vi "motion control_Z.vi"(2 "position":dbl, 3 "acceleration":dbl, 4 "maxVelocity":dbl, 5 ".NET Refnum in":refnum<k24>) -> (1 ".NET Refnum out":refnum<k24>)   [LabVIEW 2021]
uses:
  C:/Users/User/Documents/Published_files/thorlabs_files/ThorLabs.MotionControl.KCube.DCServoCLI.dll
  thorlabs_files/ThorLabs.MotionControl.KCube.DCServoCLI.dll
  <vilib>/ptbypt/NI_PtbyPt.lvlib
panel:
  out "end":bool=TRUE
  out "x < y?":bool
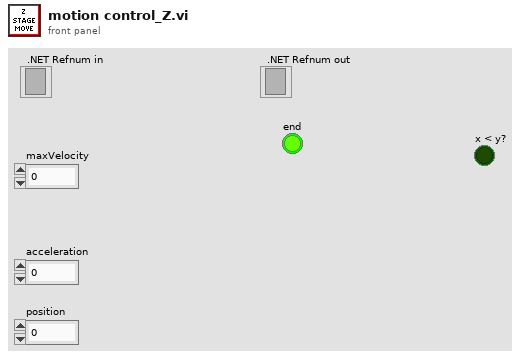
[diagram p1: front panel]
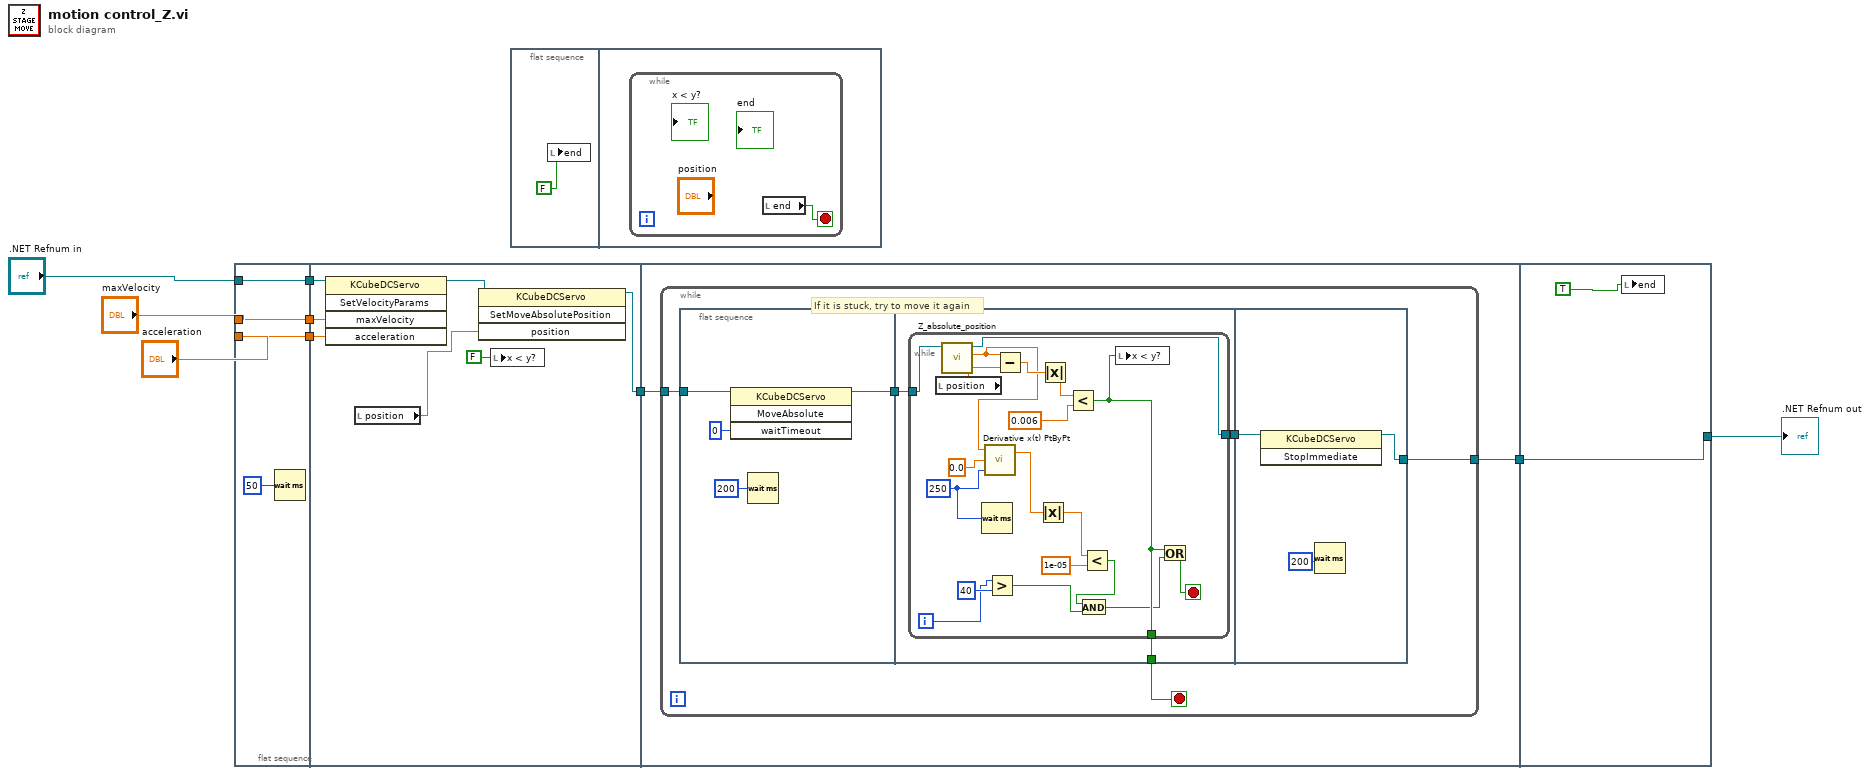
[diagram p0: block diagram]
diagram:
  n1 = flat-sequence {
    tunnel: "maxVelocity" -> [w11]
    tunnel: "acceleration" -> [w12]
    tunnel: ".NET Refnum in" -> [w13]
    tunnel: [w13] -> w3
    tunnel: [w12] -> w2
    tunnel: [w11] -> w1
    tunnel: [w14] -> w6
    tunnel: w3 -> [w20]
    tunnel: w2 -> [w19]
    tunnel: w1 -> [w18]
    tunnel: w6 -> [w22]
    tunnel: [w21] -> w4
    tunnel: [w57] -> w5
    tunnel: w4 -> [w57]
    frame #0 {
      n2 = Wait (ms)(milliseconds to wait=u32 50) -> ()  [unwired: 1 out]
    }
    frame #1 {
      n3 = invoke class="KCubeDCServo" method="SetVelocityParams"(reference=w20, "maxVelocity"=w18, "acceleration"=w19) -> (reference out=w17:refnum<k24>)  [unwired: 2 in, 4 out]
      n4 = local read "position"() -> (w15:dbl)
      n5 = invoke class="KCubeDCServo" method="SetMoveAbsolutePosition"(reference=w17, "position"=w15) -> (reference out=w14:refnum<k24>)  [unwired: 2 in, 3 out]
      n6 = local write "x < y?"(FALSE ("x < y?")) -> ()
    }
    frame #2 {
      n7 = while {
        tunnel: w22 -> [w27]
        tunnel: [w24] -> w21
        stop <- w25 stop-if-true
        # "If it is stuck, try to move it again"
        n8 = flat-sequence {
          tunnel: w27 -> [w29]
          tunnel: [w28] -> w26
          tunnel: w26 -> [w34]
          tunnel: [w33] -> w25
          tunnel: [w32] -> w23
          tunnel: w23 -> [w56]
          tunnel: [w55] -> w24
          frame #0 {
            n9 = invoke class="KCubeDCServo" method="MoveAbsolute"(reference=w29, "waitTimeout"=0) -> (reference out=w28:refnum<k24>)  [unwired: 2 in, 3 out]
            n10 = Wait (ms)(milliseconds to wait=u32 200) -> ()  [unwired: 1 out]
          }
          frame #1 {
            n11 = while {
              tunnel: w34 -> [w53]
              tunnel: [w40] -> w33
              tunnel: [w37] -> w32
              i -> [w43]
              stop <- w38 stop-if-true
              w48 = u32 250 ("milliseconds to wait")
              n12 = local read "position"() -> (w50:dbl)
              n13 = call "Z_absolute_position.vi"(".NET Refnum in"=w53) -> ("Numeric"=w46:dbl, ".NET Refnum out"=w37:refnum<k24>)  [unwired: 9 in]
              n14 = Wait (ms)(milliseconds to wait=w48) -> ()  [unwired: 1 out]
              n15 = call <vilib>:"Derivative x(t) PtByPt.vi"("dt"=w48, "initial condition"=0.0, "x"=w46) -> ("dx/dt"=w36:dbl)  [unwired: 1 in, 1 out]
              n16 = Greater?(x=w43, y=40) -> (0:w42:bool)
              n17 = Subtract(x=w46, y=w50) -> (x-y=w52:dbl)
              n18 = Absolute Value(x=w36) -> (abs(x)=w35:dbl)
              n19 = Absolute Value(x=w52) -> (abs(x)=w51:dbl)
              n20 = Less?(x=w51, y=0.006) -> (x < y?=w40:bool)
              n21 = Less?(x=w35, y=1e-05) -> (x < y?=w41:bool)
              n22 = And(x=w41, y=w42) -> (x .and. y?=w39:bool)
              n23 = local write "x < y?"(w40) -> ()
              n24 = Or(x=w40, y=w39) -> (x .or. y?=w38:bool)
            }
          }
          frame #2 {
            n25 = invoke class="KCubeDCServo" method="StopImmediate"(reference=w56) -> (reference out=w55:refnum<k24>)  [unwired: 2 in, 2 out]
            n26 = Wait (ms)(milliseconds to wait=u32 200) -> ()  [unwired: 1 out]
          }
        }
      }
    }
    frame #3 {
      n27 = local write "end"(TRUE) -> ()
    }
  }
  n28 = flat-sequence {
    frame #0 {
      n29 = local write "end"(FALSE ("end")) -> ()
    }
    frame #1 {
      n30 = while {
        stop <- w60 stop-if-true
        n31 = local read "end"() -> (w60:bool)
      }
    }
  }
  ".NET Refnum out" <- w5
